vi "Validate IP Address.vi"(10 "String":string) -> (2 "Valid IP Address?":bool)   [LabVIEW 2016]
uses:
  <vilib>/regexp/Match Regular Expression.xnode
panel:
  out "After empty?":bool
  out "Before empty?":bool
  out "after substring":string
  out "before substring":string
  out "match substring":string
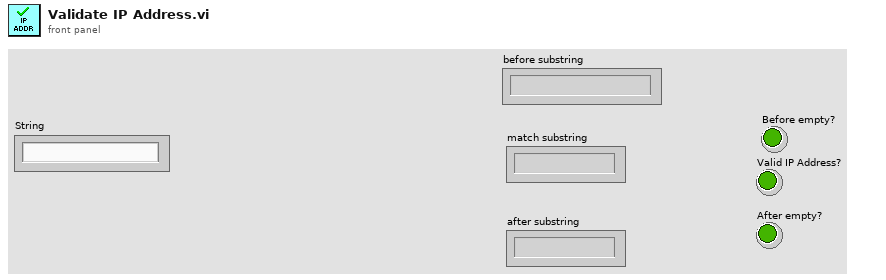
[diagram p1: front panel]
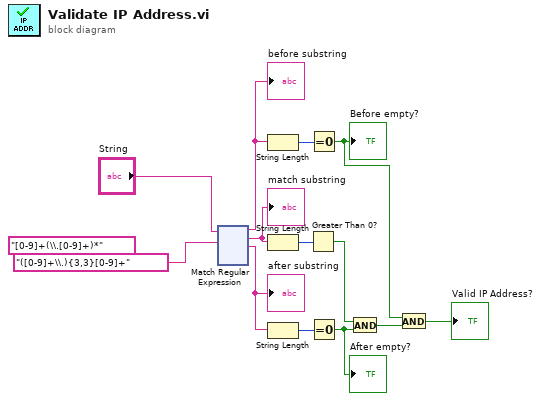
[diagram p0: block diagram]
diagram:
  (unwired) "[0-9]+(\\.[0-9]+)*" ("regular expression")
  n1 = xnode "Match Regular Expression"("input string"="String", "regular expression"="([0-9]+\\.){3,3}[0-9]+") -> ("before match"=w7:string, "whole match"=w13:string, "after match"=w6:string)  [unwired: 4 in, 2 out]
  "match substring" <- w13
  "before substring" <- w7
  "after substring" <- w6
  n2 = String Length(string=w7) -> (length=w11:i32)
  n3 = String Length(string=w13) -> (length=w12:i32)
  n4 = String Length(string=w6) -> (length=w5:i32)
  n5 = Greater Than 0?(x=w12) -> (x > 0?=w8:bool)
  n6 = Equal To 0?(x=w11) -> (x = 0?=w10:bool)
  "Before empty?" <- w10
  n7 = Equal To 0?(x=w5) -> (x = 0?=w4:bool)
  "After empty?" <- w4
  n8 = And(x=w8, y=w4) -> (x .and. y?=w9:bool)
  n9 = And(x=w10, y=w9) -> (x .and. y?=→"Valid IP Address?":bool)
